vi "Connect.vi"(6 "error in":errorcluster, 7 "Address":string, 9 "ICommHandler in":refnum<class "ICommHandler.lvclass">) -> (0 "error out":errorcluster, 3 "ICommHandler out":refnum<class "ICommHandler.lvclass">)   [LabVIEW 2021, in "wamplv.lvlib" / "ICommHandler.lvclass"]
uses:
  ICommHandler.lvclass
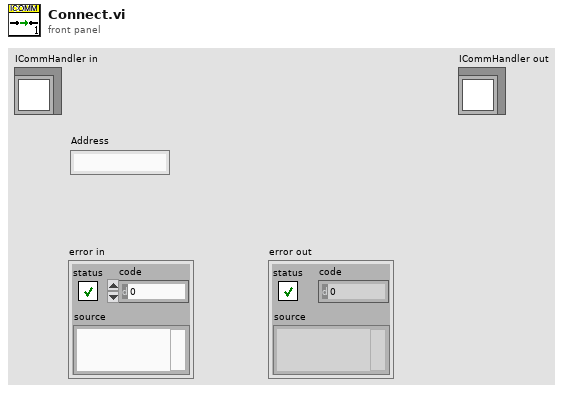
[diagram p1: front panel]
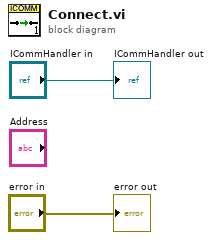
[diagram p0: block diagram]
diagram:
  "ICommHandler out" <- "ICommHandler in"
  "error out" <- "error in"
